vi "Init.vi"(8 "error in (no error)":errorcluster, 11 "Data in":refnum<class "SharedVariable_Bus.lvclass">) -> (0 "error out":errorcluster, 3 "Data out":refnum<class "SharedVariable_Bus.lvclass">)   [LabVIEW 2021, in "SharedVariable_Bus.lvclass"]
doc: "Abstract Data Classes 2.1.1.12\nTim Streeter - TSA\nCopyright (c) 2024, TSA"
uses:
  SharedVariable_Bus.lvclass
  C:/Program Files (x86)/National Instruments/LabVIEW 2021/vi.lib/TSA/Omni-Bus/Omni-Bus/Bus Access/Bus_Access.lvclass
  SharedVariable_Bus.lvclass/SharedVariable_Bus.ctl
  <vilib>/TSA/LVabs_Shared Variable/Bool/conc_SharedVar_Bool.lvclass
  C:/Program Files (x86)/National Instruments/LabVIEW 2021/vi.lib/TSA/Abstract Data Classes/Abs_Types/Value/Abs_Value.lvclass
  <vilib>/TSA/LVabs_Shared Variable/STR/conc_SharedVar_STR.lvclass
  <vilib>/TSA/LVabs_Shared Variable/Var/conc_SharedVar_Var.lvclass
  <vilib>/TSA/LVabs_Shared Variable/WFM/conc_SharedVar_WFM.lvclass
  <vilib>/TSA/LVabs_Shared Variable/Time/conc_SharedVar_Time.lvclass
  <vilib>/TSA/LVabs_Shared Variable/DBL/conc_SharedVar_DBL.lvclass
  <vilib>/TSA/LVabs_Shared Variable/SGL/conc_SharedVar_SGL.lvclass
  <vilib>/TSA/LVabs_Shared Variable/I8/conc_SharedVar_I8.lvclass
  <vilib>/TSA/LVabs_Shared Variable/I16/conc_SharedVar_I16.lvclass
  <vilib>/TSA/LVabs_Shared Variable/I32/conc_SharedVar_I32.lvclass
  <vilib>/TSA/LVabs_Shared Variable/I64/conc_SharedVar_I64.lvclass
  <vilib>/TSA/LVabs_Shared Variable/U8/conc_SharedVar_U8.lvclass
  <vilib>/TSA/LVabs_Shared Variable/U16/conc_SharedVar_U16.lvclass
  <vilib>/TSA/LVabs_Shared Variable/U32/conc_SharedVar_U32.lvclass
  <vilib>/TSA/LVabs_Shared Variable/U64/conc_SharedVar_U64.lvclass
  <vilib>/TSA/Omni-Bus/Omni-Bus/Bus Access/Bus_Access.lvclass/Bus_Access.ctl
  Properties/Read SV Containers.vi
  Properties/Read Add Container Name to Tag.vi
  <vilib>/TSA/Omni-Bus/Omni-Bus/Bus Access/Properties/Write Values.vi
  <vilib>/TSA/Omni-Bus/Omni-Bus/Bus Access/Properties/Write Tags.vi
  <vilib>/TSA/Abstract Data Classes/Abs_Types/Value/Abs_Value.lvclass
  C:/Program Files (x86)/National Instruments/LabVIEW 2021/vi.lib/TSA/Abstract Data Classes/Abs_Types/Type/Abs_Type.lvclass
  <vilib>/TSA/LVabs_Shared Variable/Bool/Initialise.vi
  <vilib>/TSA/LVabs_Shared Variable/STR/Initialise.vi
  <vilib>/TSA/LVabs_Shared Variable/Var/Initialise.vi
  <vilib>/TSA/LVabs_Shared Variable/WFM/Initialise.vi
  <vilib>/TSA/LVabs_Shared Variable/Time/Initialise.vi
  <vilib>/TSA/LVabs_Shared Variable/DBL/Initialise.vi
  <vilib>/TSA/LVabs_Shared Variable/SGL/Initialise.vi
  <vilib>/TSA/LVabs_Shared Variable/I8/Initialise.vi
  <vilib>/TSA/LVabs_Shared Variable/I16/Initialise.vi
  <vilib>/TSA/LVabs_Shared Variable/I32/Initialise.vi
  <vilib>/TSA/LVabs_Shared Variable/I64/Initialise.vi
  <vilib>/TSA/LVabs_Shared Variable/U8/Initialise.vi
  <vilib>/TSA/LVabs_Shared Variable/U16/Initialise.vi
  <vilib>/TSA/LVabs_Shared Variable/U32/Initialise.vi
  <vilib>/TSA/LVabs_Shared Variable/U64/Initialise.vi
  <resource>/objmgr/ni.var.rc
  <vilib>/Utility/Data Type/NI_Data Type.lvlib
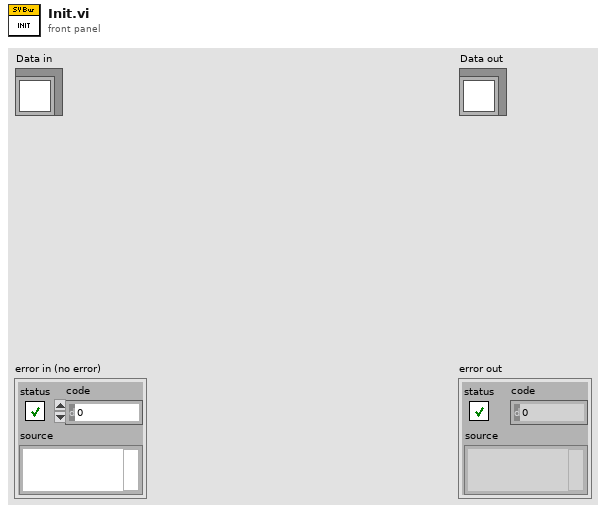
[diagram p1: front panel]
types:
  T1 = typedef "NI_Data Type.lvlib/Data Type.ctl" = enum8{"Invalid Type", "Void", "I8", "I16", "I32", "I64", "U8", "U16", "U32", "U64", "Single Float", "Double Float", "Extended Float", "Single Complex", "Double Complex", "Extended Complex", "Enum U8", "Enum U16", "Enum U32", "Enum U64", "Single Float With Unit", "Double Float With Unit", "Extended Float With Unit", "Single Complex with Unit", "Double Complex with Unit", "Extended Complex with Unit", "Boolean", "String", "Path", "Picture", "Tag", "Array", "Cluster", "Variant", "LV Variant", "Waveform", "Timestamp", "Digital Waveform", "Digital Data", "ExpressData", "Refnum", "External Data", "VI", "Poly VI", "LabVIEW Class Instance", "Fixed Point", "Set Collection", "Map Collection"}
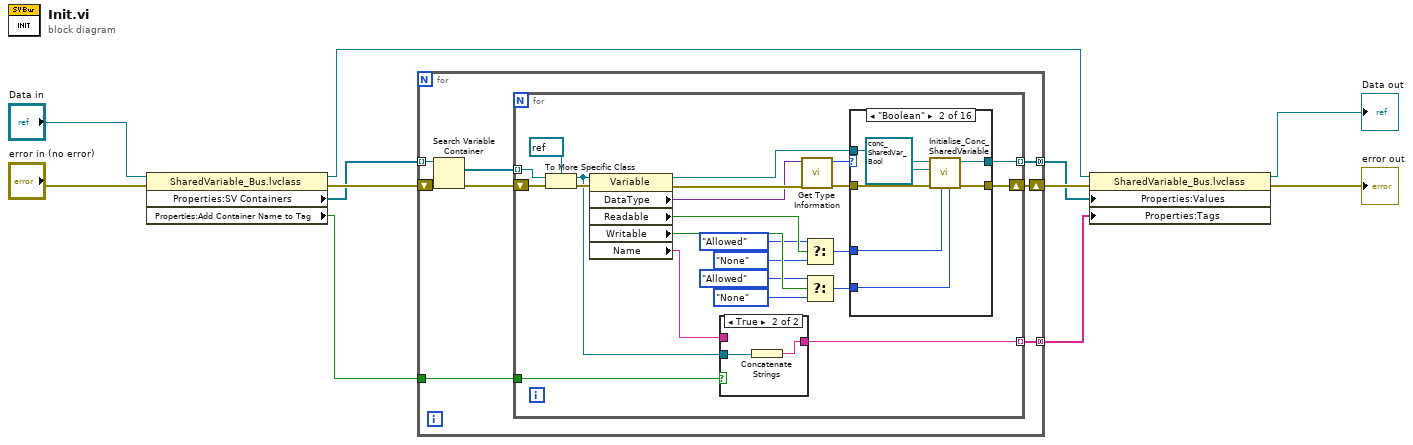
[diagram p0: block diagram]
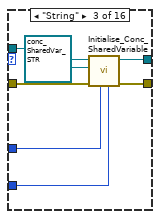
[diagram p4: hidden frame]
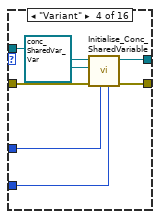
[diagram p5: hidden frame]
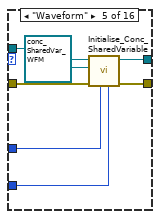
[diagram p6: hidden frame]
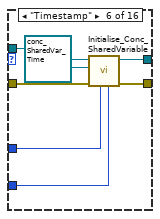
[diagram p7: hidden frame]
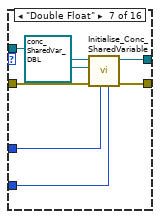
[diagram p8: hidden frame]
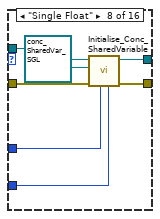
[diagram p9: hidden frame]
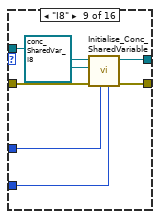
[diagram p10: hidden frame]
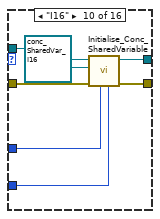
[diagram p11: hidden frame]
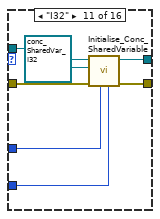
[diagram p12: hidden frame]
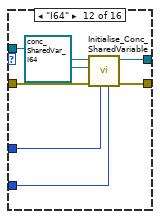
[diagram p13: hidden frame]
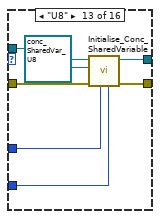
[diagram p14: hidden frame]
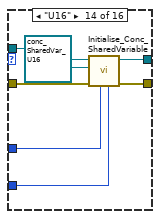
[diagram p15: hidden frame]
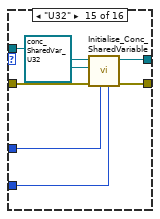
[diagram p16: hidden frame]
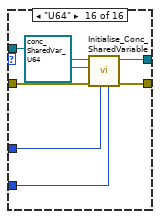
[diagram p17: hidden frame]
diagram:
  n1 = property class="SharedVariable_Bus.lvclass"(reference="Data in", error in="error in (no error)") -> (reference out=w4:refnum<class "SharedVariable_Bus.lvclass">, error out=w9:errorcluster, "Properties:SV Containers"=w2:refnum<k21>[], "Properties:Add Container Name to Tag"=w1:bool)
  n2 = for {
    tunnel: w2 -> [w18] mode=indexing
    tunnel: [w14] -> w7 mode=concatenating
    tunnel: [w13] -> w6 mode=concatenating
    shift-right: [w15] -> w8
    shift-left: w9 -> [w19]
    tunnel: w1 -> [w12]
    n3 = Search Variable Container(8:w19, 11:w18) -> (0:w17:errorcluster, 2:w16:refnum<k21>[])  [unwired: 4 in, 1 out]
    n4 = for {
      tunnel: w16 -> [w39] mode=indexing
      shift-right: [w34] -> w15
      shift-left: w17 -> [w41]
      tunnel: [w33] -> w14 mode=indexing
      tunnel: [w22] -> w13 mode=indexing
      tunnel: w12 -> [w20]
      n5 = To More Specific Class(target class=refnum<k21> refnum ("shared variable refnum in"), reference=w39, error in=w41) -> (specific class reference=w21:refnum<k21>, error out=w40:errorcluster)
      n6 = property class="Variable"(reference=w21, error in=w40) -> (reference out=w32:refnum<k21>, error out=w38:errorcluster, "DataType"=w37:variant, "Readable"=w31:bool, "Writable"=w30:bool, "Name"=w23:string)
      n7 = case shown="True" w20 {
        tunnel: w23 -> [w43 _]
        tunnel: [w43 w45] -> w22
        tunnel: w21 -> [_ w44]
        frame False {
        }
        frame True {
          n8 = Concatenate Strings(w44) -> (w45:string)
        }
      }
      n9 = call <vilib>:"Get Type Information.vi"("error in (no error)"=w38, "variant"=w37) -> ("error out"=w35:errorcluster, "type"=w36:T1)  [unwired: 5 in, 3 out]
      n10 = Select(t=enum8{"Allowed", "Required", "None"}."Allowed" ("Read Access"), s=w31, f=enum8{"Allowed", "Required", "None"}."None" ("Read Access")) -> (s? t:f=w25:enum8{"Allowed", "Required", "None"})
      n11 = Select(t=enum8{"Allowed", "Required", "None"}."Allowed" ("Read Access"), s=w30, f=enum8{"Allowed", "Required", "None"}."None" ("Read Access")) -> (s? t:f=w24:enum8{"Allowed", "Required", "None"})
      n12 = case shown="\"Boolean\"" w36 {
        tunnel: w35 -> [w46 w53 w60 w67 w74 w81 w88 w95 w102 w109 w116 w123 w130 w137 w144 w151]
        tunnel: [w46 w52 w59 w66 w73 w80 w87 w94 w101 w108 w115 w122 w129 w136 w143 w150] -> w34
        tunnel: [_ w51 w58 w65 w72 w79 w86 w93 w100 w107 w114 w121 w128 w135 w142 w149] -> w33
        tunnel: w32 -> [_ w50 w57 w64 w71 w78 w85 w92 w99 w106 w113 w120 w127 w134 w141 w148]
        tunnel: w25 -> [_ w49 w56 w63 w70 w77 w84 w91 w98 w105 w112 w119 w126 w133 w140 w147]
        tunnel: w24 -> [_ w48 w55 w62 w69 w76 w83 w90 w97 w104 w111 w118 w125 w132 w139 w146]
        frame Default {
        }
        frame "Boolean" {
          n13 = call-poly <vilib>:"Initialise_Conc_SharedVariable.vi"("Write Access"=w48, "Read Access"=w49, "error in (no error)"=w53, "shared variable refnum"=w50, "abs_SharedVar_Bool in"=refnum<class "conc_SharedVar_Bool.lvclass"> refnum) -> ("error out"=w52:errorcluster, "abs_SharedVar_Bool out"=w51:refnum<class "conc_SharedVar_Bool.lvclass">)  [unwired: 5 in]
        }
        frame "String" {
          n14 = call-poly <vilib>:"Initialise_Conc_SharedVariable.vi"("Write Access"=w55, "Read Access"=w56, "error in (no error)"=w60, "shared variable refnum"=w57, "abs_SharedVar_Bool in"=refnum<class "conc_SharedVar_STR.lvclass"> refnum) -> ("error out"=w59:errorcluster, "abs_SharedVar_Bool out"=w58:refnum<class "conc_SharedVar_STR.lvclass">)  [unwired: 5 in]
        }
        frame "Variant" {
          n15 = call-poly <vilib>:"Initialise_Conc_SharedVariable.vi"("Write Access"=w62, "Read Access"=w63, "error in (no error)"=w67, "shared variable refnum"=w64, "abs_SharedVar_Bool in"=refnum<class "conc_SharedVar_Var.lvclass"> refnum) -> ("error out"=w66:errorcluster, "abs_SharedVar_Bool out"=w65:refnum<class "conc_SharedVar_Var.lvclass">)  [unwired: 5 in]
        }
        frame "Waveform" {
          n16 = call-poly <vilib>:"Initialise_Conc_SharedVariable.vi"("Write Access"=w69, "Read Access"=w70, "error in (no error)"=w74, "shared variable refnum"=w71, "abs_SharedVar_Bool in"=refnum<class "conc_SharedVar_WFM.lvclass"> refnum) -> ("error out"=w73:errorcluster, "abs_SharedVar_Bool out"=w72:refnum<class "conc_SharedVar_WFM.lvclass">)  [unwired: 5 in]
        }
        frame "Timestamp" {
          n17 = call-poly <vilib>:"Initialise_Conc_SharedVariable.vi"("Write Access"=w76, "Read Access"=w77, "error in (no error)"=w81, "shared variable refnum"=w78, "abs_SharedVar_Bool in"=refnum<class "conc_SharedVar_Time.lvclass"> refnum) -> ("error out"=w80:errorcluster, "abs_SharedVar_Bool out"=w79:refnum<class "conc_SharedVar_Time.lvclass">)  [unwired: 5 in]
        }
        frame "Double Float" {
          n18 = call-poly <vilib>:"Initialise_Conc_SharedVariable.vi"("Write Access"=w83, "Read Access"=w84, "error in (no error)"=w88, "shared variable refnum"=w85, "abs_SharedVar_Bool in"=refnum<class "conc_SharedVar_DBL.lvclass"> refnum) -> ("error out"=w87:errorcluster, "abs_SharedVar_Bool out"=w86:refnum<class "conc_SharedVar_DBL.lvclass">)  [unwired: 5 in]
        }
        frame "Single Float" {
          n19 = call-poly <vilib>:"Initialise_Conc_SharedVariable.vi"("Write Access"=w90, "Read Access"=w91, "error in (no error)"=w95, "shared variable refnum"=w92, "abs_SharedVar_Bool in"=refnum<class "conc_SharedVar_SGL.lvclass"> refnum) -> ("error out"=w94:errorcluster, "abs_SharedVar_Bool out"=w93:refnum<class "conc_SharedVar_SGL.lvclass">)  [unwired: 5 in]
        }
        frame "I8" {
          n20 = call-poly <vilib>:"Initialise_Conc_SharedVariable.vi"("Write Access"=w97, "Read Access"=w98, "error in (no error)"=w102, "shared variable refnum"=w99, "abs_SharedVar_Bool in"=refnum<class "conc_SharedVar_I8.lvclass"> refnum) -> ("error out"=w101:errorcluster, "abs_SharedVar_Bool out"=w100:refnum<class "conc_SharedVar_I8.lvclass">)  [unwired: 5 in]
        }
        frame "I16" {
          n21 = call-poly <vilib>:"Initialise_Conc_SharedVariable.vi"("Write Access"=w104, "Read Access"=w105, "error in (no error)"=w109, "shared variable refnum"=w106, "abs_SharedVar_Bool in"=refnum<class "conc_SharedVar_I16.lvclass"> refnum) -> ("error out"=w108:errorcluster, "abs_SharedVar_Bool out"=w107:refnum<class "conc_SharedVar_I16.lvclass">)  [unwired: 5 in]
        }
        frame "I32" {
          n22 = call-poly <vilib>:"Initialise_Conc_SharedVariable.vi"("Write Access"=w111, "Read Access"=w112, "error in (no error)"=w116, "shared variable refnum"=w113, "abs_SharedVar_Bool in"=refnum<class "conc_SharedVar_I32.lvclass"> refnum) -> ("error out"=w115:errorcluster, "abs_SharedVar_Bool out"=w114:refnum<class "conc_SharedVar_I32.lvclass">)  [unwired: 5 in]
        }
        frame "I64" {
          n23 = call-poly <vilib>:"Initialise_Conc_SharedVariable.vi"("Write Access"=w118, "Read Access"=w119, "error in (no error)"=w123, "shared variable refnum"=w120, "abs_SharedVar_Bool in"=refnum<class "conc_SharedVar_I64.lvclass"> refnum) -> ("error out"=w122:errorcluster, "abs_SharedVar_Bool out"=w121:refnum<class "conc_SharedVar_I64.lvclass">)  [unwired: 5 in]
        }
        frame "U8" {
          n24 = call-poly <vilib>:"Initialise_Conc_SharedVariable.vi"("Write Access"=w125, "Read Access"=w126, "error in (no error)"=w130, "shared variable refnum"=w127, "abs_SharedVar_Bool in"=refnum<class "conc_SharedVar_U8.lvclass"> refnum) -> ("error out"=w129:errorcluster, "abs_SharedVar_Bool out"=w128:refnum<class "conc_SharedVar_U8.lvclass">)  [unwired: 5 in]
        }
        frame "U16" {
          n25 = call-poly <vilib>:"Initialise_Conc_SharedVariable.vi"("Write Access"=w132, "Read Access"=w133, "error in (no error)"=w137, "shared variable refnum"=w134, "abs_SharedVar_Bool in"=refnum<class "conc_SharedVar_U16.lvclass"> refnum) -> ("error out"=w136:errorcluster, "abs_SharedVar_Bool out"=w135:refnum<class "conc_SharedVar_U16.lvclass">)  [unwired: 5 in]
        }
        frame "U32" {
          n26 = call-poly <vilib>:"Initialise_Conc_SharedVariable.vi"("Write Access"=w139, "Read Access"=w140, "error in (no error)"=w144, "shared variable refnum"=w141, "abs_SharedVar_Bool in"=refnum<class "conc_SharedVar_U32.lvclass"> refnum) -> ("error out"=w143:errorcluster, "abs_SharedVar_Bool out"=w142:refnum<class "conc_SharedVar_U32.lvclass">)  [unwired: 5 in]
        }
        frame "U64" {
          n27 = call-poly <vilib>:"Initialise_Conc_SharedVariable.vi"("Write Access"=w146, "Read Access"=w147, "error in (no error)"=w151, "shared variable refnum"=w148, "abs_SharedVar_Bool in"=refnum<class "conc_SharedVar_U64.lvclass"> refnum) -> ("error out"=w150:errorcluster, "abs_SharedVar_Bool out"=w149:refnum<class "conc_SharedVar_U64.lvclass">)  [unwired: 5 in]
        }
      }
    }
  }
  n28 = property class="SharedVariable_Bus.lvclass"(reference=w4, error in=w8, "Properties:Values"=w7, "Properties:Tags"=w6) -> (reference out=→"Data out":refnum<class "SharedVariable_Bus.lvclass">, error out=→"error out":errorcluster)
